vi "IMAQ HL-Grab.vi"(8 "ErrIn":errorcluster, 11 "IF Name":string="img0") -> (0 "ErrOut":errorcluster, 3 "ImgOut":T1)   [LabVIEW 2013]
doc: "Use this template to build a VI to use as a subVI."
uses:
  <vilib>/vision/Image Controls.llb/IMAQ Image.ctl
panel:
  in  "stop":bool
  out "Frame Rate":dbl(knob) scale=0.0..100.0
  # "Input Parameters"
  # "Output Parameters"
  # "VI Description:\nThis VI is created to Grab a image from imaging device."
  # ":: MVI Framework V1.0 ::\nAuthor:Gaoke Yang\nEmail: gaoke.yang@yahoo.com\nWeb: www.mvicontrol.com\nCopyright (C) 2013, MVI Technologies All Rights Reserved"
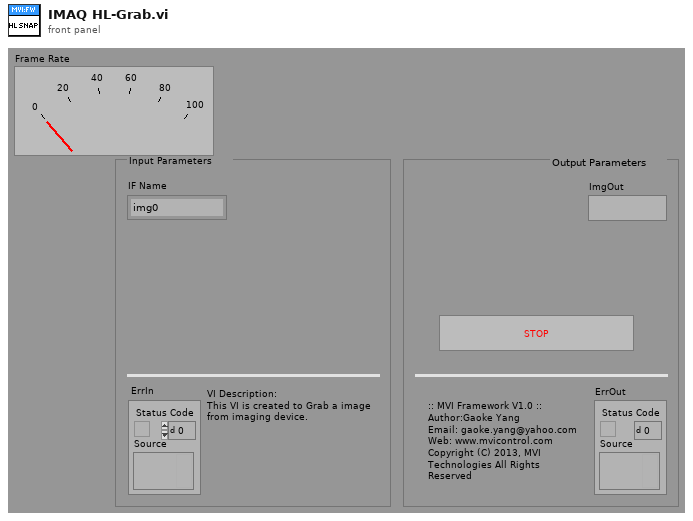
[diagram p1: front panel]
types:
  T1 = typedef "IMAQ Image.ctl" = refnum<image>
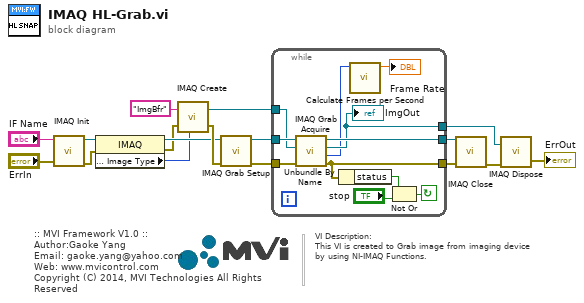
[diagram p0: block diagram]
diagram:
  # "VI Description:\nThis VI is created to Grab image from imaging device\nby using NI-IMAQ Functions."
  # ":: MVI Framework V1.0 ::\nAuthor:Gaoke Yang\nEmail: gaoke.yang@yahoo.com\nWeb: www.mvicontrol.com\nCopyright (C) 2014, MVI Technologies All Rights Reserved"
  n1 = call <vilib>:"IMAQ Init.vi"("error in (no error)"="ErrIn", "Interface Name"="IF Name") -> ("error out"=w7:errorcluster, "IMAQ Session Out"=w8:refnum<k11>)  [unwired: 8 out]
  n2 = property class="IMAQ"(reference=w8, error in=w7) -> (reference out=w6:refnum<k11>, error out=w5:errorcluster, "Image Parameters : Image Type"=w4:u32)
  n3 = call "IMAQ Create"("Image Name"="ImgBfr", "Image Type"=w4, "error in (no error)"=w5) -> ("New Image"=w13:T1, "error out"=w14:errorcluster)  [unwired: 1 in, 1 out]
  n4 = call <vilib>:"IMAQ Grab Setup.vi"("error in (no error)"=w14, "IMAQ Session In"=w6) -> ("error out"=w11:errorcluster, "IMAQ Session Out"=w12:refnum<k11>)  [unwired: 8 out]
  n5 = while {
    tunnel: [w22] -> w9
    tunnel: w13 -> [w26]
    tunnel: w12 -> [w27]
    tunnel: w11 -> [w28]
    tunnel: [w21] -> w3
    tunnel: [w20] -> w1
    stop <- w24 continue-if-true
    n6 = call <vilib>:"IMAQ Grab Acquire.vi"("error in (no error)"=w28, "Image In"=w26, "IMAQ Session In"=w27) -> ("error out"=w21:errorcluster, "Acquired Buffer Number"=w19:u32, "Image Out"=w20:T1, "IMAQ Session Out"=w22:refnum<k11>)  [unwired: 1 in, 4 out]
    "ImgOut" <- w20
    n7 = Unbundle By Name(w21) -> ("status"=w25:bool)
    n8 = call <vilib>:"Calculate Frames per Second.vi"("Buffer Number"=w19) -> ("Acquired Frames/s"=→"Frame Rate":dbl)  [unwired: 8 in, 2 out]
    n9 = Not Or(1:"stop", 2:w25) -> (0:w24:bool)
  }
  n10 = call <vilib>:"IMAQ Close.vi"("error in (no error)"=w3, "IMAQ Session In"=w9) -> ("error out"=w2:errorcluster)  [unwired: 9 out]
  n11 = call "IMAQ Dispose"("Image"=w1, "error in (no error)"=w2) -> ("error out"=→"ErrOut":errorcluster)  [unwired: 1 in, 3 out]
